vi "Can Edit Type.vi"(11 "Type Descriptor":T1={"Name"="", "Direction"=enum."Sink", "Value Type"=enum."Bool", "Default"=variant, "Terminal Mode"=enum."Recommended", "Min"=variant, "Max"=variant, "Step"=variant, "Options"=[], "Terminal Type"=enum."Unwired", "Type Mode"=enum."Output", "Value Mode"=enum."Basic"}) -> (3 "Can Edit?":bool)   [LabVIEW 2020, in "Parallel Diagram Block.xnode"]
uses:
  Parallel Diagram Block.xnode
  Parallel Block/Type Descriptor.ctl
  Parallel Block/Direction.ctl
  Parallel Block/Value Type.ctl
  Parallel Block/Terminal Mode.ctl
  Parallel Block/Terminal Type.ctl
  Parallel Block/Parallel Block.lvlib
  Parallel Block/Type Mode.ctl
  Parallel Block/Value Mode.ctl
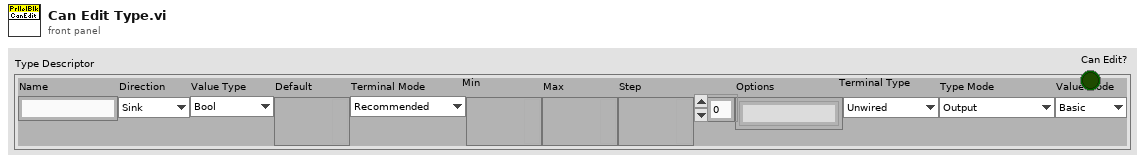
[diagram p1: front panel]
types:
  T1 = typedef "Parallel Block.lvlib/Type Descriptor.ctl" = cluster{"Name":string, "Direction":T2, "Value Type":T3, "Default":variant, "Terminal Mode":T4, "Min":variant, "Max":variant, "Step":variant, "Options":string[], "Terminal Type":T5, "Type Mode":T6, "Value Mode":T7}
  T2 = typedef "Parallel Block.lvlib/Direction.ctl" = enum16{"Sink", "Source"}
  T3 = typedef "Parallel Block.lvlib/Value Type.ctl" = enum16{"Unknown", "Bool", "U8", "U16", "U32", "U64", "I8", "I16", "I32", "I64", "SGL", "DBL", "CSG", "CDB", "CDBWfm", "String", "DBLWfm"}
  T4 = typedef "Parallel Block.lvlib/Terminal Mode.ctl" = enum16{"Recommended", "Required", "None"}
  T5 = typedef "Parallel Block.lvlib/Terminal Type.ctl" = enum16{"Unwired", "BadType", "Connection", "Value", "Control Ref", "BadRefType"}
  T6 = typedef "Parallel Block.lvlib/Type Mode.ctl" = enum16{"Output", "Adaptive (Lossy)", "Strict (Lossy)", "Lossless"}
  T7 = typedef "Parallel Block.lvlib/Value Mode.ctl" = enum16{"Basic", "Range", "Select"}
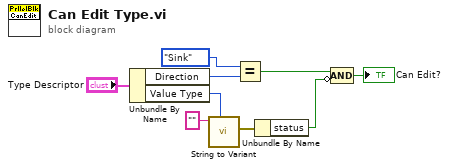
[diagram p0: block diagram]
diagram:
  n1 = Unbundle By Name("Type Descriptor") -> ("Direction"=w5:T2, "Value Type"=w8:T3)
  n2 = call "String to Variant.vi"("Value Type"=w8, "String"="") -> ("error out"=w6:errorcluster)  [unwired: 7 in, 2 out]
  n3 = Equal?(x=Direction."Sink", y=w5) -> (x = y?=w2:bool)
  n4 = Unbundle By Name(w6) -> ("status"=w3:bool)
  n5 = Compound Arithmetic op=AND(w2, invert w3) -> (→"Can Edit?":bool)
